vi "setModulation.vi"(0 "Interface in":T2, 5 "modulationConfig":T1, 11 "error in (no error)":errorcluster) -> (4 "Interface out":T2, 15 "error out":errorcluster)   [LabVIEW 2017, in "BuckBoostInterface.lvlib"]
uses:
  BuckBoostInterface.lvlib
  Interface.ctl
  <instrlib>/_niInstr/Instruction Framework/v1/Host/Instruction Target/niInstr Instruction Target v1 Host.lvclass
  <instrlib>/_niInstr/Instruction Framework/v1/Host/Instruction Framework Context/niInstr Instruction Framework Context v1 Host.lvclass
  modulationConfig.ctl
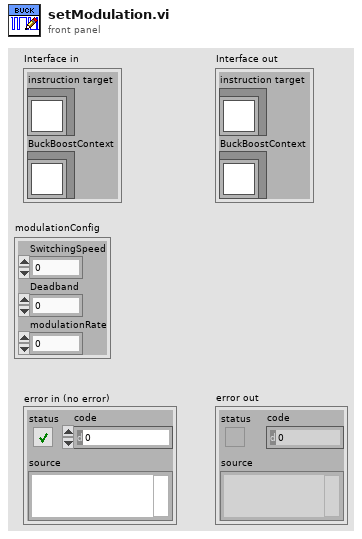
[diagram p1: front panel]
types:
  T1 = typedef "BuckBoostInterface.lvlib/modulationConfig.ctl" = cluster{"SwitchingSpeed":dbl, "Deadband":dbl, "modulationRate":dbl}
  T2 = typedef "BuckBoostInterface.lvlib/Interface.ctl" = cluster{"instruction target":refnum<class "niInstr Instruction Target v1 Host.lvclass">, "BuckBoostContext":refnum<class "niInstr Instruction Framework Context v1 Host.lvclass">}
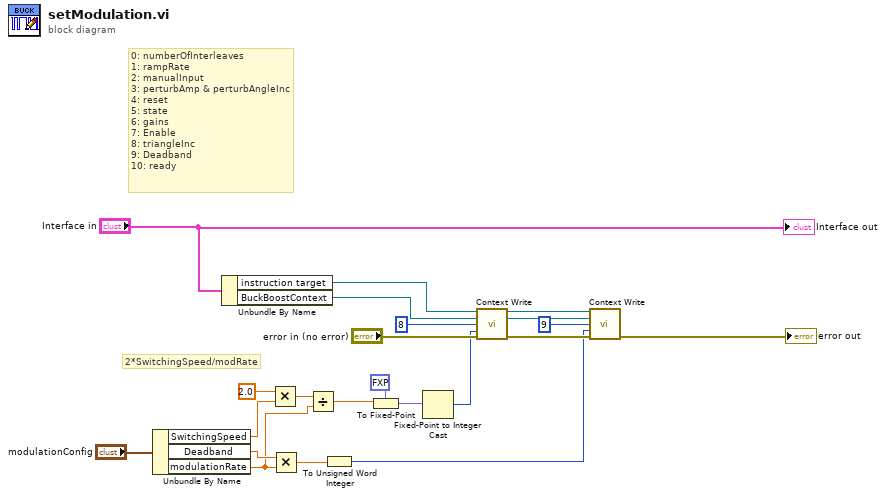
[diagram p0: block diagram]
diagram:
  # "2*SwitchingSpeed/modRate"
  # "0: numberOfInterleaves\n1: rampRate\n2: manualInput\n3: perturbAmp & perturbAngleInc\n4: reset\n5: state\n6: gains\n7: Enable\n8: triangleInc\n9: Deadband\n10: ready"
  n1 = Unbundle By Name("modulationConfig") -> ("SwitchingSpeed"=w9:dbl, "Deadband"=w12:dbl, "modulationRate"=w6:dbl)
  n2 = Unbundle By Name("Interface in") -> ("instruction target"=w20:refnum<class "niInstr Instruction Target v1 Host.lvclass">, "BuckBoostContext"=w19:refnum<class "niInstr Instruction Framework Context v1 Host.lvclass">)
  n3 = Multiply(x=2.0, y=w9) -> (x*y=w7:dbl)
  n4 = Multiply(x=w12, y=w6) -> (x*y=w11:dbl)
  n5 = Divide(x=w7, y=w6) -> (x/y=w4:dbl)
  n6 = To Unsigned Word Integer(number=w11) -> (unsigned 16bit integer=w10:u16)
  n7 = To Fixed-Point(fixed-point type=fxp<+,18,0> 0.0 ("Data"), number=w4) -> (fixed-point=w3:fxp<+,18,0>)
  n8 = Fixed-Point to Integer Cast(1:w3) -> (0:w2:u32)
  n9 = call <instrlib>:"Context Write.vi"("instruction target in"=w20, "context in"=w19, "address"=u64 8, "data"=w2, "error in"="error in (no error)") -> ("instruction target out"=w17:refnum<class "niInstr Instruction Target v1 Host.lvclass">, "context out"=w15:refnum<class "niInstr Instruction Framework Context v1 Host.lvclass">, "error out"=w16:errorcluster)  [unwired: 8 in]
  n10 = call <instrlib>:"Context Write.vi"("instruction target in"=w17, "context in"=w15, "address"=u64 9, "data"=w10, "error in"=w16) -> ("error out"=→"error out":errorcluster)  [unwired: 8 in, 2 out]
  "Interface out" <- "Interface in"
